vi "AssembleBLMultiplotScript-Profiles.vi"(0 "gnuplotIn":string, 1 "lambdaBounds":T1={"Min"={"Auto"=FALSE, "Value"=0.0}, "Max"={"Auto"=FALSE, "Value"=0.6}}, 3 "sigma/U bounds":T1={"Min"={"Auto"=FALSE, "Value"=0.0}, "Max"={"Auto"=FALSE, "Value"=0.12}}, 5 "ProfileFilename":string="profile.dat", 7 "Mapping":enum8{"Lin", "Log"}(ring)=enum."Log", 9 "HeightAxisBounds":T1={"Min"={"Auto"=FALSE, "Value"=5.0}, "Max"={"Auto"=FALSE, "Value"=2000.0}}, 11 "jitterFraction":dbl=0.03, 12 "U/UrefBounds":T1={"Min"={"Auto"=FALSE, "Value"=0.0}, "Max"={"Auto"=FALSE, "Value"=1.2}}, 14 "TI bounds":T1={"Min"={"Auto"=FALSE, "Value"=0.0}, "Max"={"Auto"=FALSE, "Value"=30.0}}) -> (4 "gnuplotOut":string)   [LabVIEW 2013]
uses:
  minAndMax.ctl
  AutoManualNumber.ctl
  margins.ctl
  axisName.ctl
  ticsAndGrids.ctl
  tics.ctl
  grids.ctl
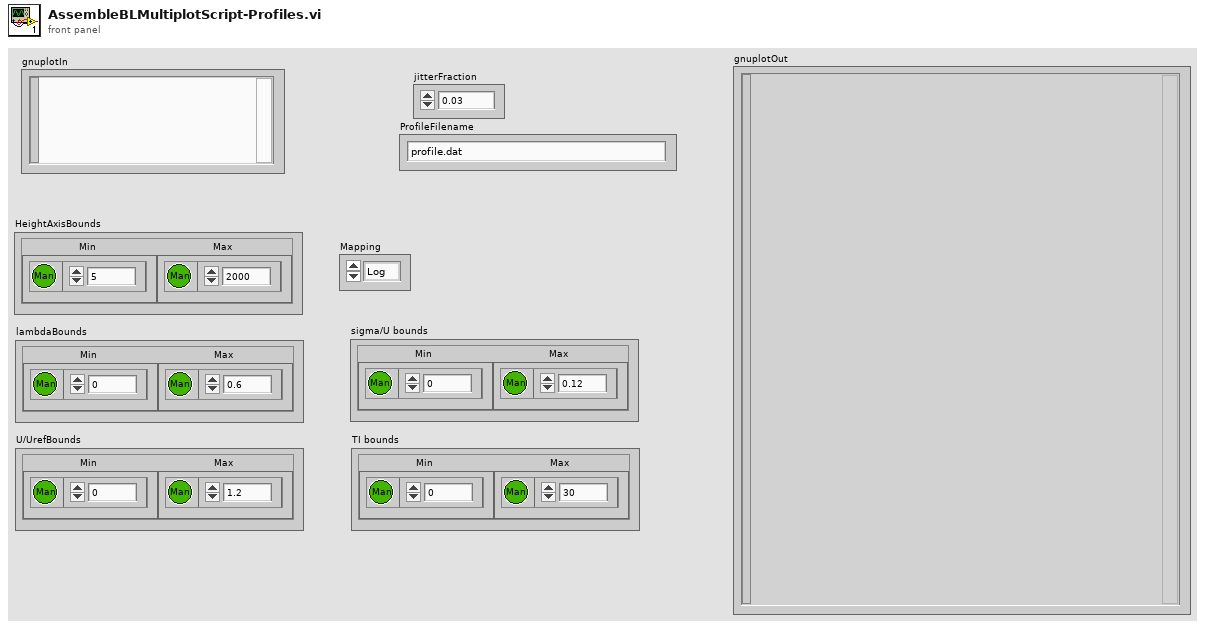
[diagram p1: front panel]
types:
  T1 = typedef "minAndMax.ctl" = cluster{"Min":T2, "Max":T2}
  T2 = typedef "AutoManualNumber.ctl" = cluster{"Auto":bool, "Value":dbl}
  T3 = typedef "ticsAndGrids.ctl" = cluster{"tics":T4, "Grids":T5, "Mapping":enum8{"Lin", "Log"}}
  T4 = typedef "tics.ctl" = cluster{"ticMin":dbl, "ticStep":dbl, "ticMax":dbl, "minorDivsPerMajor":i32, "ticSpacing":enum16{"Auto Tics", "Fixed spacing", "Fixed Minimum and Spacing", "Start, Spacing and Maximum", "Approx n Tics (rounded)"}, "ticPosition":enum16{"Inside, no mirror", "Inside, mirrored", "Outside, no mirror", "Outside, mirrored", "Invisible"}}
  T5 = typedef "grids.ctl" = cluster{"Gridlines":enum16{"No grids", "Major grid", "Minor grid", "Major and Minor"}, "Zeroaxis":enum16{"No zero axis", "Show zero axis"}}
  T6 = typedef "axisName.ctl" = string
  T7 = typedef "margins.ctl" = cluster{"Top":dbl, "Bottom":dbl, "Left":dbl, "Right":dbl}
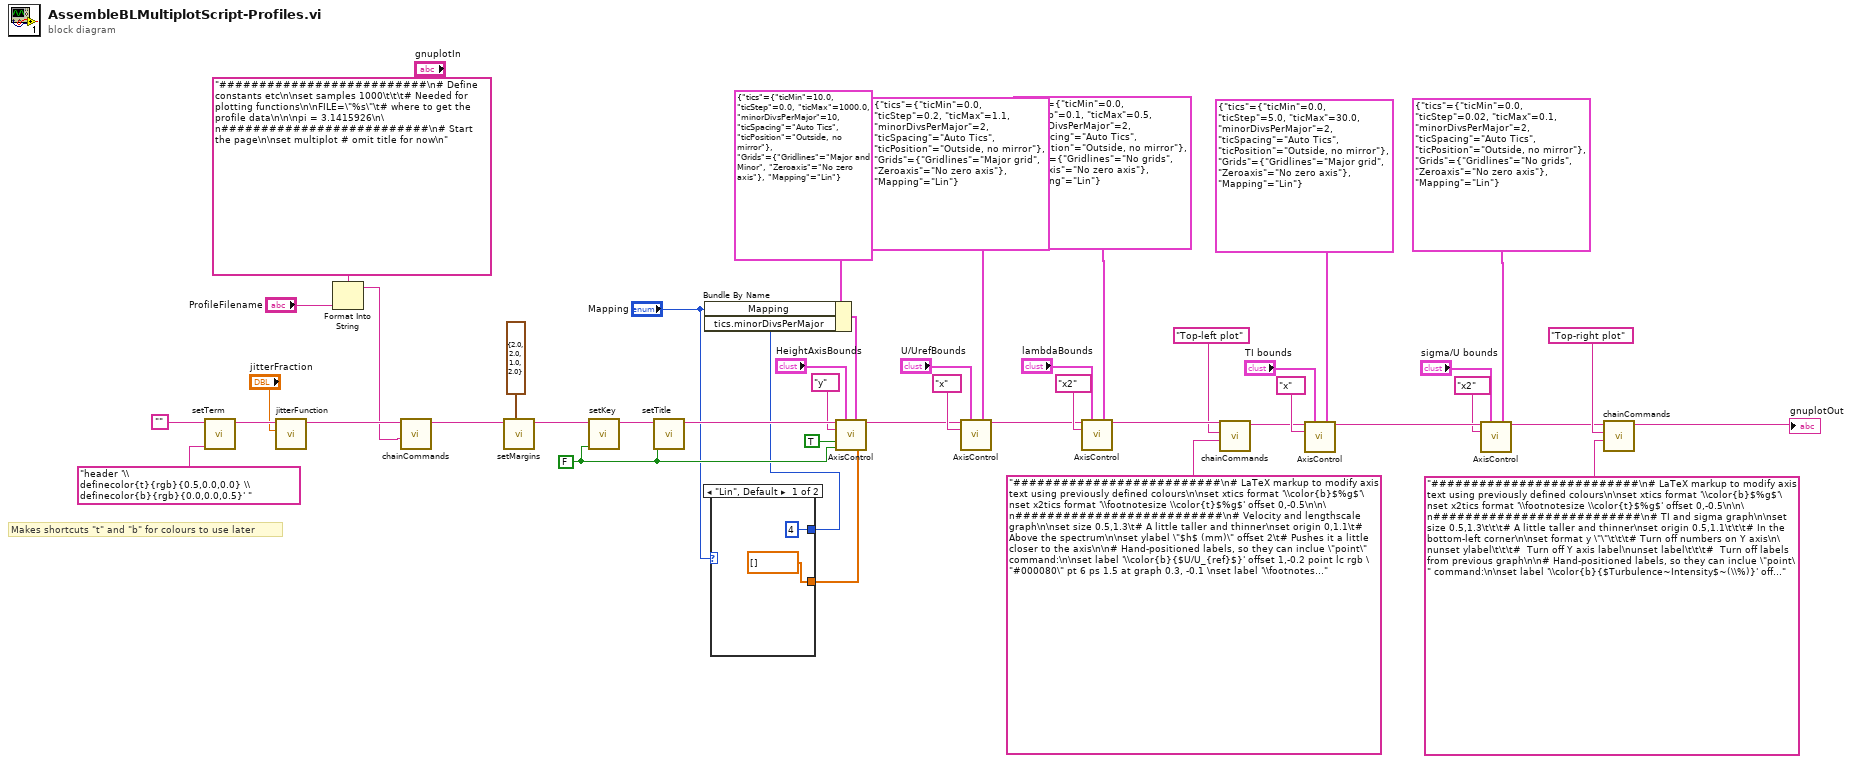
[diagram p0: block diagram]
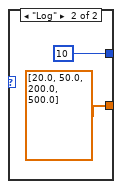
[diagram p2: hidden frame]
diagram:
  w32 = FALSE ("Set?")
  # "Makes shortcuts \"t\" and \"b\" for colours to use later"
  n1 = call "setTerm.vi"("Additional Terminal Options"="header '\\definecolor{t}{rgb}{0.5,0.0,0.0} \\definecolor{b}{rgb}{0.0,0.0,0.5}' ", "String in"="") -> ("String out"=w43:string)  [unwired: 8 in, 1 out]
  n2 = call "jitterFunction.vi"("jitterFraction"="jitterFraction", "String in"=w43) -> ("String out"=w23:string)  [unwired: 8 in, 1 out]
  n3 = Format Into String(format string="##########################\n# Define constants etc\n\nset samples 1000\t\t\t# Needed for plotting functions\n\nFILE=\"%s\"\t# where to get the profile data\n\n\npi = 3.1415926\n\n##########################\n# Start the page\n\nset multiplot # omit title for now\n" ("Command"), "ProfileFilename") -> (resulting string=w15:string)  [unwired: 2 in, 1 out]
  n4 = call "chainCommands.vi"("Command"=w15, "StringIn"=w23) -> ("StringOut"=w22:string)  [unwired: 9 in]
  n5 = call "setMargins.vi"("Margins"=T7 {"Top"=2.0, "Bottom"=2.0, "Left"=1.0, "Right"=2.0}, "String in"=w22) -> ("String out"=w40:string)  [unwired: 8 in, 1 out]
  n6 = call "setKey.vi"("Set?"=w32, "String in"=w40) -> ("String out"=w39:string)  [unwired: 8 in, 1 out]
  n7 = call "setTitle.vi"("Set?"=w32, "String in"=w39) -> ("String out"=w38:string)  [unwired: 8 in, 1 out]
  n8 = case shown="\"Lin\", Default" "Mapping" {
    tunnel: [dbl[] [] ("AdditionalTics") dbl[] [20.0, 50.0, 200.0, 500.0] ("AdditionalTics")] -> w31
    tunnel: [4 ("minorDivsPerMajor") 10 ("minorDivsPerMajor")] -> w1
    frame "Lin", Default {
    }
    frame "Log" {
    }
  }
  n9 = Bundle By Name(cluster=T3 {"tics"={"ticMin"=10.0, "ticStep"=0.0, "ticMax"=1000.0, "minorDivsPerMajor"=10, "ticSpacing"=enum."Auto Tics", "ticPosition"=enum."Outside, no mirror"}, "Grids"={"Gridlines"=enum."Major and Minor", "Zeroaxis"=enum."No zero axis"}, "Mapping"=enum."Lin"} ("ticsAndGrids"), "Mapping"="Mapping", "tics.minorDivsPerMajor"=w1) -> (w34:T3)
  n10 = call "AxisControl.vi"("String in"=w38, "AxisBounds"="HeightAxisBounds", "ticsAndGrids"=w34, "Axis"=T6 "y", "ShowNumbers?"=TRUE, "ShowLabel?"=w32, "AdditionalTics"=w31) -> ("String out"=w27:string)  [unwired: 7 in, 1 out]
  n11 = call "AxisControl.vi"("String in"=w27, "AxisBounds"="U/UrefBounds", "ticsAndGrids"=T3 {"tics"={"ticMin"=0.0, "ticStep"=0.2, "ticMax"=1.1, "minorDivsPerMajor"=2, "ticSpacing"=enum."Auto Tics", "ticPosition"=enum."Outside, no mirror"}, "Grids"={"Gridlines"=enum."Major grid", "Zeroaxis"=enum."No zero axis"}, "Mapping"=enum."Lin"}, "Axis"=T6 "x") -> ("String out"=w26:string)  [unwired: 10 in, 1 out]
  n12 = call "AxisControl.vi"("String in"=w26, "AxisBounds"="lambdaBounds", "ticsAndGrids"=T3 {"tics"={"ticMin"=0.0, "ticStep"=0.1, "ticMax"=0.5, "minorDivsPerMajor"=2, "ticSpacing"=enum."Auto Tics", "ticPosition"=enum."Outside, no mirror"}, "Grids"={"Gridlines"=enum."No grids", "Zeroaxis"=enum."No zero axis"}, "Mapping"=enum."Lin"}, "Axis"=T6 "x2") -> ("String out"=w18:string)  [unwired: 10 in, 1 out]
  n13 = call "chainCommands.vi"("Command"="##########################\n# LaTeX markup to modify axis text using previously defined colours\n\nset xtics format '\\color{b}$%g$'\nset x2tics format '\\footnotesize \\color{t}$%g$' offset 0,-0.5\n\n\n##########################\n# Velocity and lengthscale graph\n\nset size 0.5,1.3\t# A little taller and thinner\nset origin 0,1.1\t# Above the spectrum\n\nset ylabel \"$h$ (mm)\" offset 2\t# Pushes it a little closer to the axis\n\n# Hand-positioned labels, so they can inclue \"point\" command:\n\nset label '\\color{b}{$U/U_{ref}$}' offset 1,-0.2 point lc rgb \"#000080\" pt 6 ps 1.5 at graph 0.3, -0.1 \nset label '\\footnotesize \\color{t}{$\\lambda(U)$ (m)}' offset 1,-0.2 point lc rgb \"#800000\" pt 2 ps 0.8 at graph 0.4, 1.08\n\n\nplot FILE index 0 using 1:(jittered($2)) axes x1y1 title 'Velocity' w points lc rgb \"#000080\" pt 6 ps 1.5, \\\nFILE index 1 using 1:(jittered($2)) axes x2y1 title 'Lengthscale' w points lc rgb \"#800000\" pt 2 ps 0.8\n\n", "Comments"="Top-left plot", "StringIn"=w18) -> ("StringOut"=w6:string)  [unwired: 8 in]
  n14 = call "AxisControl.vi"("String in"=w6, "AxisBounds"="TI bounds", "ticsAndGrids"=T3 {"tics"={"ticMin"=0.0, "ticStep"=5.0, "ticMax"=30.0, "minorDivsPerMajor"=2, "ticSpacing"=enum."Auto Tics", "ticPosition"=enum."Outside, no mirror"}, "Grids"={"Gridlines"=enum."Major grid", "Zeroaxis"=enum."No zero axis"}, "Mapping"=enum."Lin"}, "Axis"=T6 "x") -> ("String out"=w9:string)  [unwired: 10 in, 1 out]
  n15 = call "AxisControl.vi"("String in"=w9, "AxisBounds"="sigma/U bounds", "ticsAndGrids"=T3 {"tics"={"ticMin"=0.0, "ticStep"=0.02, "ticMax"=0.1, "minorDivsPerMajor"=2, "ticSpacing"=enum."Auto Tics", "ticPosition"=enum."Outside, no mirror"}, "Grids"={"Gridlines"=enum."No grids", "Zeroaxis"=enum."No zero axis"}, "Mapping"=enum."Lin"}, "Axis"=T6 "x2") -> ("String out"=w4:string)  [unwired: 10 in, 1 out]
  n16 = call "chainCommands.vi"("Command"="##########################\n# LaTeX markup to modify axis text using previously defined colours\n\nset xtics format '\\color{b}$%g$'\nset x2tics format '\\footnotesize \\color{t}$%g$' offset 0,-0.5\n\n\n##########################\n# TI and sigma graph\n\nset size 0.5,1.3\t\t\t# A little taller and thinner\nset origin 0.5,1.1\t\t\t# In the bottom-left corner\n\nset format y \"\"\t\t\t# Turn off numbers on Y axis\n\nunset ylabel\t\t\t#  Turn off Y axis label\nunset label\t\t\t#  Turn off labels from previous graph\n\n# Hand-positioned labels, so they can inclue \"point\" command:\n\nset label '\\color{b}{$Turbulence~Intensity$~(\\%)}' offset 1,-0.2 point lc rgb \"#000080\" pt 6 ps 1.5 at graph 0.15, -0.1\n\nset label '\\footnotesize \\color{t}{$\\sigma(U)/U_{ref}$}' offset 1,-0.2 point lc rgb \"#800000\" pt 2 ps 0.8 at graph 0.35, 1.08\n\n\nplot FILE index 2 using 1:(jittered($2)) axes x1y1 title 'Turbulence' w points lc rgb '#000080' pt 6 ps 1.5, \\\nFILE index 3 using 1:(jittered($2)) axes x2y1 title 'sigma/U' w points lc rgb '#800000' pt 2 ps 0.8\n\nunset multiplot\t# All done :-)", "Comments"="Top-right plot", "StringIn"=w4) -> ("StringOut"=→"gnuplotOut":string)  [unwired: 8 in]
